vi "Main.vi"(8 "error in":errorcluster, 11 "TopUI in":refnum<class "TopUI.lvclass">) -> (0 "error out":errorcluster, 3 "TopUI out":refnum<class "TopUI.lvclass">)   [LabVIEW 2025, in "TopUI.lvclass"]
doc: "The <b>Queued Message Handler</b> of the Worker that owns this VI."
uses:
  TopUI.lvclass
  C:/Program Files (x86)/National Instruments/LabVIEW 2025/vi.lib/addons/_Workers/Library/Classes/Worker/Worker.lvclass
  TopUI.lvclass/TopUI.ctl
  Initialization Data.ctl
  Response Cases.ctl
  rql_WriteSetupParameter.ctl
  rql_ReadWaveformData.ctl
  <vilib>/addons/_Workers/Library/Classes/Message Queue/Message Queue.lvclass
  Oscilloscope/Oscilloscope.lvclass
panel:
  out "OscillscopeType":string
  out "Waveform Graph":waveform(dbl)(graph)
  in  "GetWaveform":bool
  in  "Setup":bool
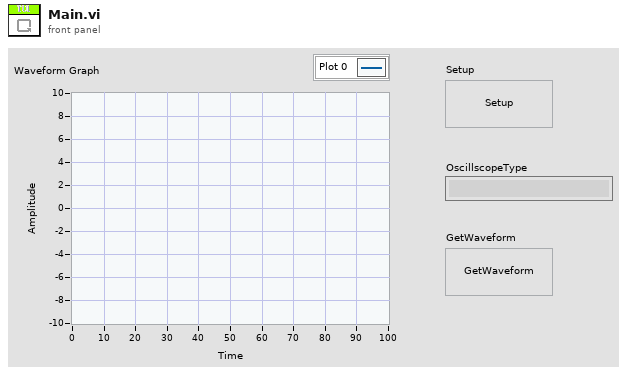
[diagram p1: front panel]
types:
  T1 = typedef "TopUI.lvclass/Initialization Data.ctl" = cluster{"Response Cases":T2}
  T2 = typedef "TopUI.lvclass/Response Cases.ctl" = cluster{"Placeholder - Can be deleted":string}
  T3 = typedef "TopUI.lvclass/rql_WriteSetupParameter.ctl" = cluster{"String":string}
  T4 = typedef "TopUI.lvclass/rql_ReadWaveformData.ctl" = cluster{"String":string}
  T5 = typedef "Oscilloscope.lvclass/rwr_WriteScopeSetup Reply.ctl" = cluster{"String":string}
  T6 = typedef "Oscilloscope.lvclass/rsp_WaveformDataRuturn.ctl" = cluster{"String":string, "Waveform":waveform(dbl)}
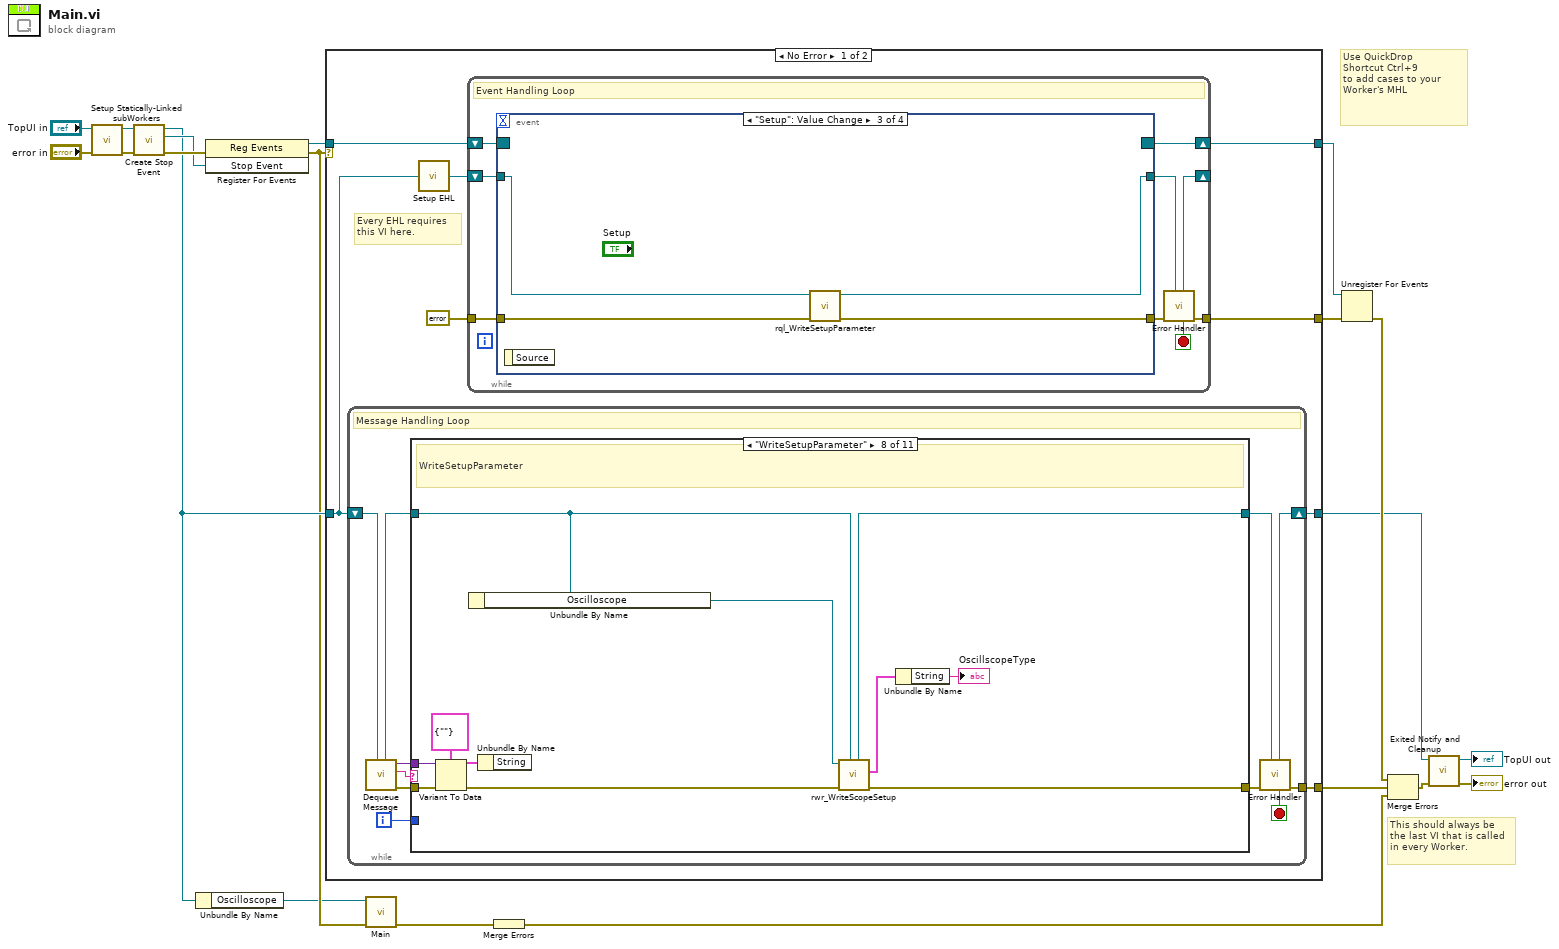
[diagram p0: block diagram]
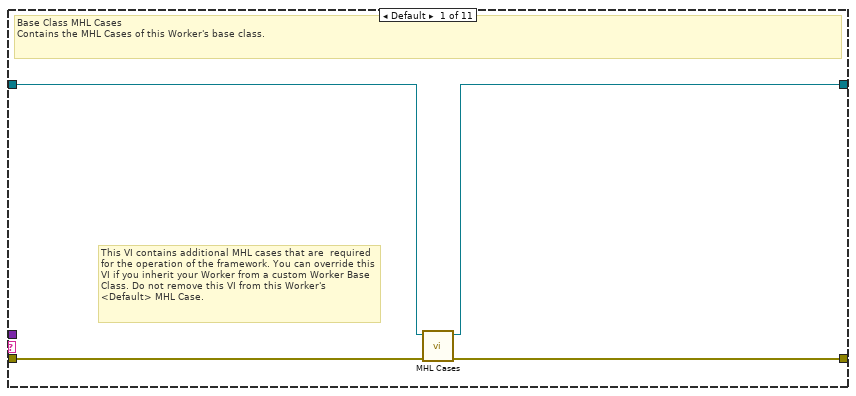
[diagram p2: hidden frame]
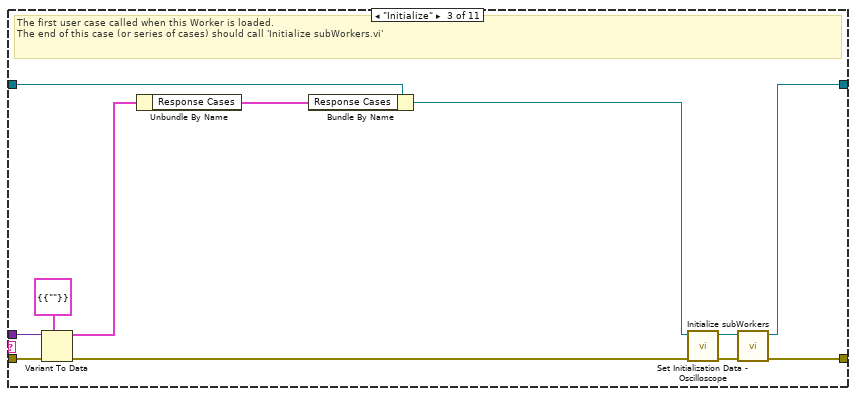
[diagram p4: hidden frame]
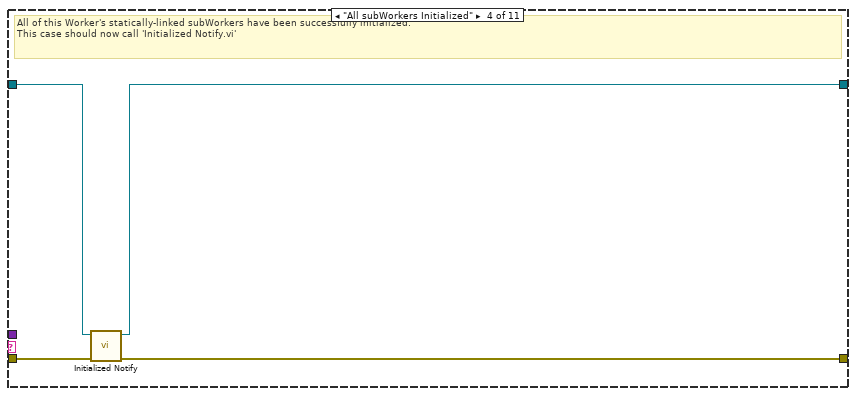
[diagram p5: hidden frame]
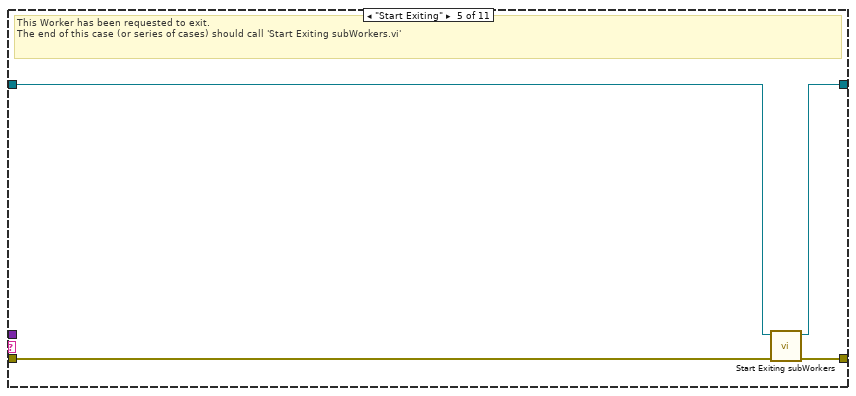
[diagram p6: hidden frame]
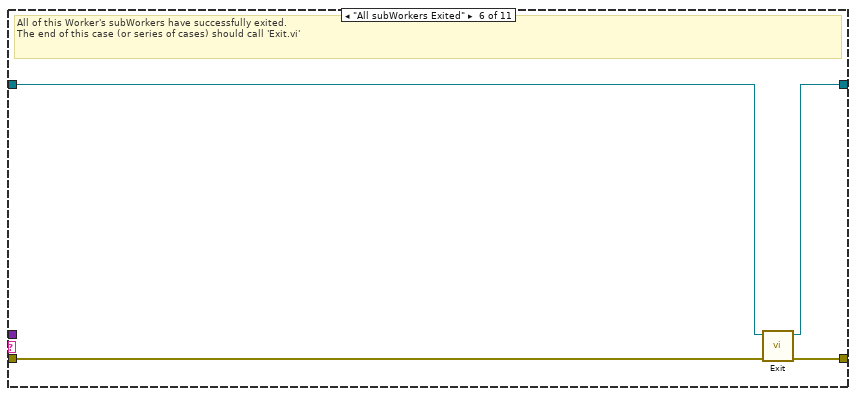
[diagram p7: hidden frame]
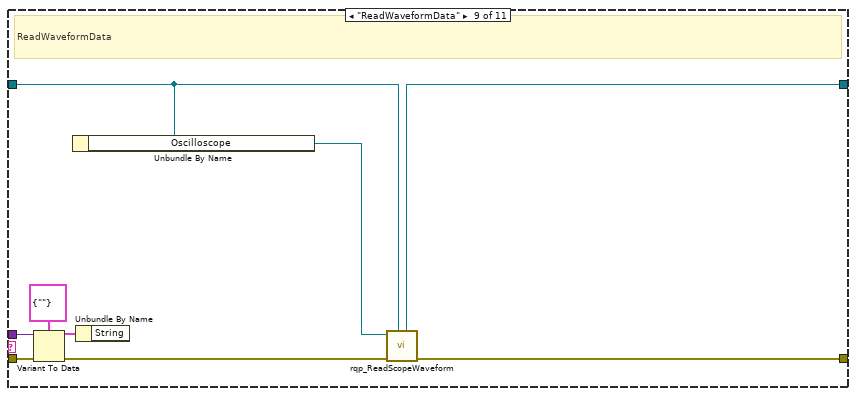
[diagram p9: hidden frame]
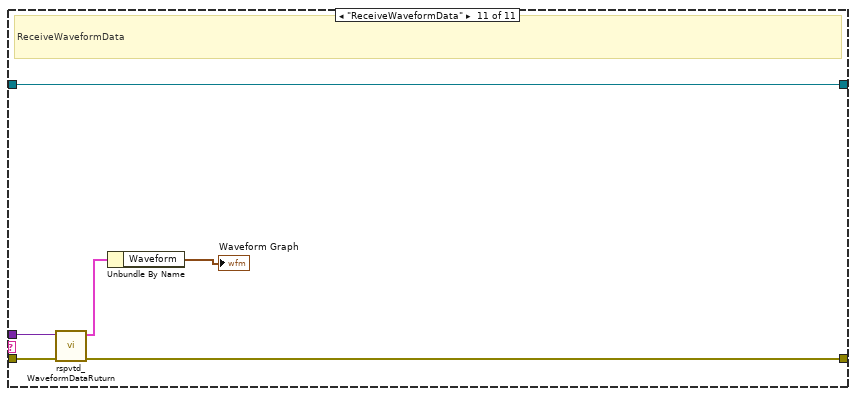
[diagram p11: hidden frame]
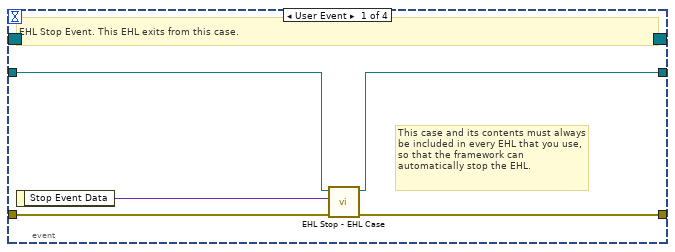
[diagram p12: hidden frame]
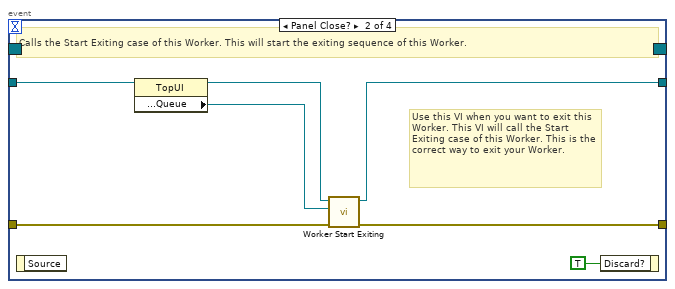
[diagram p13: hidden frame]
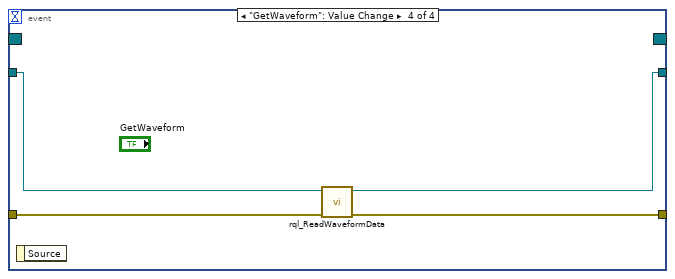
[diagram p14: hidden frame]
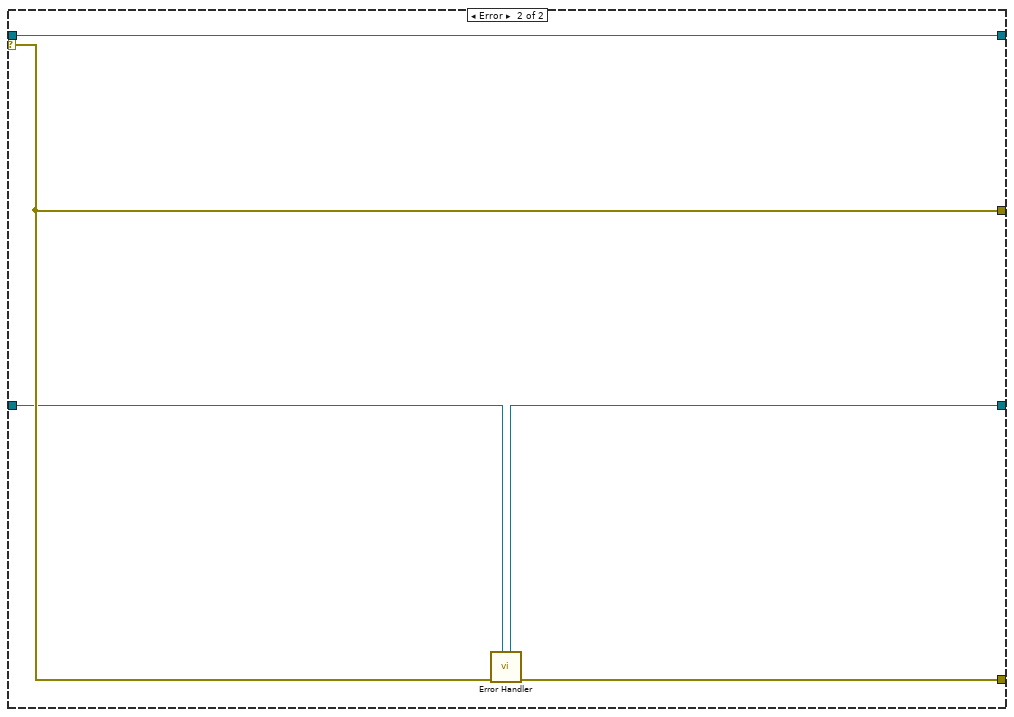
[diagram p15: hidden frame]
diagram:
  # "Use QuickDrop\nShortcut Ctrl+9\nto add cases to your\nWorker's MHL"
  # "This should always be the last VI that is called in every Worker."
  n1 = call "Setup Statically-Linked subWorkers.vi"("error in"="error in", "TopUI in"="TopUI in") -> ("error out"=w6:errorcluster, "TopUI out"=w4:refnum<class "TopUI.lvclass">)  [unwired: 8 in]
  n2 = call-dynamic "Create Stop Event.vi"("error in"=w6, "Worker"=w4) -> ("error out"=w15:errorcluster, "Stop Event"=w12:refnum<user-event>, "Worker out"=w9:refnum<class "TopUI.lvclass">)  [unwired: 7 in]
  n3 = Unbundle By Name(w9) -> ("Oscilloscope"=w1:refnum<class "Oscilloscope.lvclass">)
  n4 = register-events(error in=w15, w12) -> (reference out=w14:refnum<event-registration>, error out=w7:errorcluster)  [unwired: 1 in]
  n5 = case shown="No Error" w7 {
    tunnel: w9 -> [w23 w130]
    tunnel: [w21 w131] -> w13
    tunnel: w14 -> [w28 w132]
    tunnel: [w25 w133] -> w19
    tunnel: [w27 w132] -> w18
    tunnel: [w22 w129] -> w16
    selector: w7 -> [_ w133]
    frame No Error {
      # "Every EHL requires\nthis VI here."
      n6 = while {
        shift-right: [w37] -> w22
        shift-left: w23 -> [w39]
        tunnel: [w38] -> w21
        i -> [w30]
        stop <- w31 stop-if-true
        # "Message Handling Loop"
        n7 = call-dynamic "Dequeue Message.vi"("Worker"=w39) -> ("error out"=w36:errorcluster, "Case out"=w32:string, "Data out"=w29:variant, "Worker out"=w34:refnum<class "TopUI.lvclass">)  [unwired: 6 in, 1 out]
        n8 = case "Worker MHL Case Structure (DO NOT CHANGE LABEL NAME)" shown="\"WriteSetupParameter\"" w32 {
          tunnel: w36 -> [w43 w44 w55 w59 w62 w69 w71 w82 w91 w93 w99]
          tunnel: [w42 w44 w57 w58 w65 w68 w71 w77 w86 w93 w97] -> w35
          tunnel: w34 -> [w41 w45 w54 w61 w63 w67 w70 w75 w84 w92 w98]
          tunnel: [w40 w45 w56 w60 w64 w66 w70 w76 w85 w92 w98] -> w33
          tunnel: w30 -> [_ _ _ _ _ _ _ _ _ _ _]
          tunnel: w29 -> [_ _ w52 _ _ _ _ w79 w88 _ w96]
          frame Default {
            # "This VI contains additional MHL cases that are  required for the operation of the framework. You can override this VI if you inherit your Worker from a custom Worker Base Class. Do not remove this VI from this Worker's <Default> MHL Case."
            # "Base Class MHL Cases\nContains the MHL Cases of this Worker's base class."
            n9 = call-dynamic "MHL Cases.vi"("error in"=w43, "Worker in"=w41) -> ("error out"=w42:errorcluster, "Worker out"=w40:refnum<class "TopUI.lvclass">)  [unwired: 8 in]
          }
          frame "------------ FRAMEWORK CASES -----------" {
            # "Start of Workers Framework Cases"
          }
          frame "Initialize" {
            # "The first user case called when this Worker is loaded.\nThe end of this case (or series of cases) should call 'Initialize subWorkers.vi'"
            n10 = Variant To Data(error in=w55, type=T1 {"Response Cases"={"Placeholder - Can be deleted"=""}} ("Initialization Data"), Variant=w52) -> (data=w51:T1, error out=w53:errorcluster)
            n11 = Unbundle By Name(w51) -> ("Response Cases"=w50:T2)
            n12 = Bundle By Name(cluster=w54, "Response Cases"=w50) -> (w46:refnum<class "TopUI.lvclass">)
            n13 = call "Set Initialization Data - Oscilloscope.vi"("error in"=w53, "TopUI in"=w46) -> ("error out"=w48:errorcluster, "TopUI out"=w47:refnum<class "TopUI.lvclass">)  [unwired: 8 in]
            n14 = call-dynamic "Initialize subWorkers.vi"("error in"=w48, "Worker"=w47) -> ("error out"=w57:errorcluster, "dup Worker out"=w56:refnum<class "TopUI.lvclass">)  [unwired: 8 in]
          }
          frame "All subWorkers Initialized" {
            # "All of this Worker's statically-linked subWorkers have been successfully initialized.\nThis case should now call 'Initialized Notify.vi'"
            n15 = call-dynamic "Initialized Notify.vi"("error in"=w59, "Worker"=w61) -> ("error out"=w58:errorcluster, "dup Worker out"=w60:refnum<class "TopUI.lvclass">)  [unwired: 8 in]
          }
          frame "Start Exiting" {
            # "This Worker has been requested to exit. \nThe end of this case (or series of cases) should call 'Start Exiting subWorkers.vi'"
            n16 = call-dynamic "Start Exiting subWorkers.vi"("error_in"=w62, "Worker"=w63) -> ("error out"=w65:errorcluster, "dup Worker out"=w64:refnum<class "TopUI.lvclass">)  [unwired: 8 in]
          }
          frame "All subWorkers Exited" {
            # "All of this Worker's subWorkers have successfully exited. \nThe end of this case (or series of cases) should call 'Exit.vi'"
            n17 = call-dynamic "Exit.vi"("error_in"=w69, "Worker"=w67) -> ("error out"=w68:errorcluster, "dup Worker out"=w66:refnum<class "TopUI.lvclass">)  [unwired: 8 in]
          }
          frame "------------- LOCAL API CASES -------------" {
            # "Start of Workers Local API Cases"
          }
          frame "WriteSetupParameter" {
            # "WriteSetupParameter"
            n18 = Variant To Data(error in=w82, type=T3 {"String"=""} ("Data"), Variant=w79) -> (data=w78:T3, error out=w81:errorcluster)
            n19 = Unbundle By Name(w75) -> ("Oscilloscope"=w74:refnum<class "Oscilloscope.lvclass">)
            n20 = Unbundle By Name(w78) -> ()  [unwired: 1 out]
            n21 = call "rwr_WriteScopeSetup.vi"("Caller in"=w75, "error in"=w81, "Oscilloscope in"=w74) -> ("error out"=w77:errorcluster, "Reply Data out"=w73:T5, "dup Caller out"=w76:refnum<class "TopUI.lvclass">)  [unwired: 5 in, 1 out]
            n22 = Unbundle By Name(w73) -> ("String"=→"OscillscopeType":string)
          }
          frame "ReadWaveformData" {
            # "ReadWaveformData"
            n23 = Variant To Data(error in=w91, type=T4 {"String"=""} ("Data"), Variant=w88) -> (data=w87:T4, error out=w90:errorcluster)
            n24 = Unbundle By Name(w84) -> ("Oscilloscope"=w83:refnum<class "Oscilloscope.lvclass">)
            n25 = Unbundle By Name(w87) -> ()  [unwired: 1 out]
            n26 = call "rqp_ReadScopeWaveform.vi"("Caller in"=w84, "error in"=w90, "Oscilloscope in"=w83) -> ("error out"=w86:errorcluster, "dup Caller out"=w85:refnum<class "TopUI.lvclass">)  [unwired: 6 in, 1 out]
          }
          frame "------------- RESPONSE CASES --------------" {
            # "Start of Workers Response Cases"
          }
          frame "ReceiveWaveformData" {
            # "ReceiveWaveformData"
            n27 = call "rspvtd_WaveformDataRuturn.vi"("error in"=w99, "Data in"=w96) -> ("error out"=w97:errorcluster, "Data out"=w95:T6)  [unwired: 8 in]
            n28 = Unbundle By Name(w95) -> ("Waveform"=→"Waveform Graph":waveform(dbl))
          }
        }
        n29 = call-dynamic "Error Handler.vi"("Worker"=w33, "error_in"=w35) -> ("error out"=w38:errorcluster, "Stop Loop"=w31:bool, "Worker out"=w37:refnum<class "TopUI.lvclass">)  [unwired: 7 in]
      }
      n30 = call-dynamic "Setup EHL.vi"("Worker"=w23) -> ("Worker out"=w24:refnum<class "TopUI.lvclass">)  [unwired: 14 in]
      n31 = while "Event Handling Loop" {
        shift-right: [w108] -> w27
        shift-left: w28 -> [w107]
        tunnel: [w103] -> w25
        tunnel: errorcluster {"status"=FALSE, "code"=0, "source"=""} ("error constant") -> [w105]
        shift-right: [w101] -> _
        shift-left: w24 -> [w106]
        stop <- w100 stop-if-true
        # "Event Handling Loop"
        n32 = event shown="[2] \"Setup\": Value Change" {
          selector: w107 -> [_ _ _ _]
          dyn-events: [_ _ _ _] -> w108
          timeout: _ -> [_ _ _ _]
          tunnel: [w112 w119 w123 w127] -> w104
          tunnel: w105 -> [w113 w118 w124 w128]
          tunnel: w106 -> [w111 w117 w122 w126]
          tunnel: [w110 w116 w121 w125] -> w102
          event User Event {
            # "This case and its contents must always be included in every EHL that you use, so that the framework can automatically stop the EHL."
            # "EHL Stop Event. This EHL exits from this case."
            n33 = event-data() -> ("Stop Event Data"=w109:variant)  [unwired: 1 in]
            n34 = call-dynamic "EHL Stop - EHL Case.vi"("error in"=w113, "Stop Event Data"=w109, "Worker"=w111) -> ("error out"=w112:errorcluster, "Worker out"=w110:refnum<class "TopUI.lvclass">)  [unwired: 7 in]
          }
          event Panel Close? {
            # "Use this VI when you want to exit this Worker. This VI will call the Start Exiting case of this Worker. This is the correct way to exit your Worker."
            # "Calls the Start Exiting case of this Worker. This will start the exiting sequence of this Worker."
            n35 = event-data() -> ()  [unwired: 1 in, 1 out]
            n36 = property class="TopUI"(reference=w117) -> (reference out=w115:refnum<class "TopUI.lvclass">, "Accessors:Read:Public API:Queue"=w114:refnum<class "Message Queue.lvclass">)  [unwired: 1 in, 1 out]
            n37 = call-dynamic "Worker Start Exiting.vi"("error_in"=w118, "Message Queue"=w114, "Worker"=w115) -> ("error out"=w119:errorcluster, "dup Worker out"=w116:refnum<class "TopUI.lvclass">)  [unwired: 7 in]
            n38 = event-data ("Event Filter Node")("Discard?"=TRUE) -> ()  [unwired: 1 in, 1 out]
          }
          event "Setup": Value Change {
            n39 = event-data() -> ()  [unwired: 1 in, 1 out]
            n40 = call "rql_WriteSetupParameter.vi"("error in"=w124, "TopUI in"=w122) -> ("error out"=w123:errorcluster, "dup TopUI out"=w121:refnum<class "TopUI.lvclass">)  [unwired: 8 in]
          }
          event "GetWaveform": Value Change {
            n41 = event-data() -> ()  [unwired: 1 in, 1 out]
            n42 = call "rql_ReadWaveformData.vi"("error in"=w128, "TopUI in"=w126) -> ("error out"=w127:errorcluster, "dup TopUI out"=w125:refnum<class "TopUI.lvclass">)  [unwired: 8 in]
          }
        }
        n43 = call-dynamic "Error Handler.vi"("Worker"=w102, "error_in"=w104) -> ("error out"=w103:errorcluster, "Stop Loop"=w100:bool, "Worker out"=w101:refnum<class "TopUI.lvclass">)  [unwired: 7 in]
      }
    }
    frame Error {
      n44 = call-dynamic "Error Handler.vi"("Worker"=w130, "error_in"=w133) -> ("error out"=w131:errorcluster, "Worker out"=w129:refnum<class "TopUI.lvclass">)  [unwired: 7 in, 1 out]
    }
  }
  n45 = call-dynamic "Main.vi"("error in"=w7, "Oscilloscope in"=w1) -> ("error out"=w3:errorcluster)  [unwired: 8 in, 1 out]
  n46 = Merge Errors(w3) -> (w2:errorcluster)
  n47 = Unregister For Events(event registration refnum=w18, error in=w19) -> (error out=w20:errorcluster)
  n48 = Merge Errors(w20, w13, w2) -> (w17:errorcluster)
  n49 = call-dynamic "Exited Notify and Cleanup.vi"("error_in"=w17, "Worker"=w16) -> ("error out"=→"error out":errorcluster, "dup Worker out"=→"TopUI out":refnum<class "TopUI.lvclass">)  [unwired: 8 in]
